vi "Write Extinction Data.vi"(8 "error in":errorcluster, 10 "CRDS Data in":refnum<class "CRDS Data.lvclass">, 11 "CRD File Obs in":refnum<class "CRD File Obs.lvclass">) -> (0 "error out":errorcluster, 3 "CRD File Obs out":refnum<class "CRD File Obs.lvclass">)   [LabVIEW 2015, in "CRD File Obs.lvclass"]
uses:
  CRD File Obs.lvclass
  Data/Main/CRDS Data.lvclass
  Data/Main/crd_data_enum.ctl
  Data/Cell/CRDS Cell Data.lvclass/CRDS Cell Data.ctl
  File IO/Class/File Observer.lvclass/File Observer.ctl
  Data/Cell/Read extParam.vi
  File IO/Class/Read File Ref.vi
  Data/Main/Read CellData.vi
  Data/Cell/CRDS Cell Data.lvclass
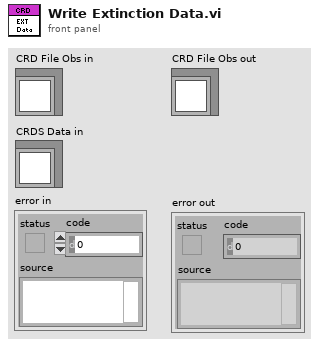
[diagram p1: front panel]
types:
  T1 = typedef "crd_data_enum.ctl" = enum8{"Time", "RHw", "TRH", "P", "Tmean", "RHsense", "TQ", "PQ", "Q", "Q0", "Qcal", "Qset", "extDilFac", "taucorr", "tau0corr", "stdevtau", "ext", "extCorr", "etau", "tau", "tau0", "Purge_Data", "NoData", "reserved", "Ttec", "Ang Exp", "Gamma", "filter", "fOverride", "notes", "max amp", "Tthermistor", "RhdilFac", "Psense", "TRHsense_bank", "RHsense_bank", "MFC_Data", "Thum", "ThumSP", "O3 Flow", "Pinlet Flow", "CLAP Flow", "O3 Add Valve", "O2 Valve", "O3 Cal"}
  T2 = enum16{"big-endian, network order", "native, host order", "little-endian"}
  T3 = typedef "extparam.ctl" = cluster{"Tau":sgl, "Tau0cor":sgl, "ext":sgl, "extCorr":sgl, "stdevTau":sgl, "eTau":sgl, "taucorr":sgl, "Tau0":sgl, "max":sgl}
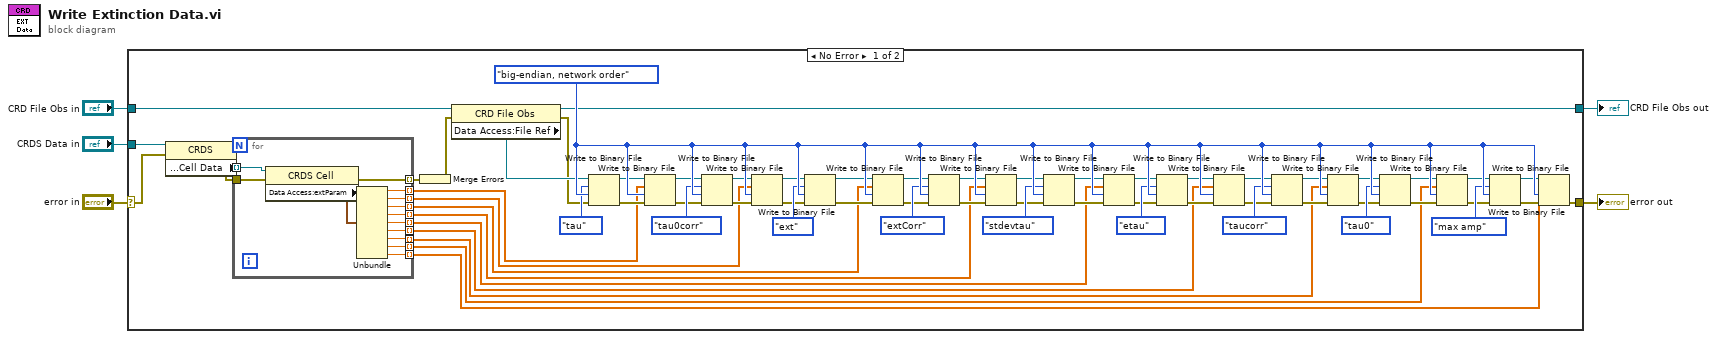
[diagram p0: block diagram]
diagram:
  n1 = case shown="No Error" "error in" {
    selector: "error in" -> [w67 w84]
    tunnel: [w7 w84] -> w4
    tunnel: [w6 w83] -> w2
    tunnel: "CRD File Obs in" -> [w11 w83]
    tunnel: "CRDS Data in" -> [w69 _]
    frame No Error {
      w65 = T2."big-endian, network order" ("byte order (0:big-endian, network order)")
      n2 = property class="CRDS"(reference=w69, error in=w67) -> (error out=w66:errorcluster, "Data Access:Cell Data"=w68:refnum<class "CRDS Cell Data.lvclass">[])  [unwired: 1 out]
      n3 = for {
        tunnel: w68 -> [w82] mode=indexing
        tunnel: w66 -> [w80]
        tunnel: [w79] -> w12 mode=indexing
        tunnel: [w78] -> w21 mode=indexing
        tunnel: [w77] -> w20 mode=indexing
        tunnel: [w76] -> w19 mode=indexing
        tunnel: [w75] -> w18 mode=indexing
        tunnel: [w74] -> w17 mode=indexing
        tunnel: [w73] -> w16 mode=indexing
        tunnel: [w72] -> w15 mode=indexing
        tunnel: [w71] -> w14 mode=indexing
        tunnel: [w70] -> w13 mode=indexing
        n4 = property class="CRDS Cell"(reference=w82, error in=w80) -> (error out=w79:errorcluster, "Data Access:extParam"=w81:T3)  [unwired: 1 out]
        n5 = Unbundle(w81) -> ("Tau"=w78:sgl, "Tau0cor"=w77:sgl, "ext"=w76:sgl, "extCorr"=w75:sgl, "stdevTau"=w74:sgl, "eTau"=w73:sgl, "taucorr"=w72:sgl, "Tau0"=w71:sgl, "max"=w70:sgl)
      }
      n6 = Merge Errors(w12) -> (w9:errorcluster)
      n7 = property class="CRD File Obs"(reference=w11, error in=w9) -> (reference out=w6:refnum<class "CRD File Obs.lvclass">, error out=w8:errorcluster, "Data Access:File Ref"=w10:refnum<file>)
      n8 = Write to Binary File(file (use dialog)=w10, data=crd_data_enum."tau" ("CRD_Data_Enum"), error in=w8, 9:w65) -> (refnum out=w42:refnum<file>, error out=w40:errorcluster)  [unwired: 2 in, 1 out]
      n9 = Write to Binary File(file (use dialog)=w42, data=w21, error in=w40, 9:w65) -> (refnum out=w43:refnum<file>, error out=w39:errorcluster)  [unwired: 2 in, 1 out]
      n10 = Write to Binary File(file (use dialog)=w43, data=crd_data_enum."tau0corr" ("CRD_Data_Enum"), error in=w39, 9:w65) -> (refnum out=w44:refnum<file>, error out=w38:errorcluster)  [unwired: 2 in, 1 out]
      n11 = Write to Binary File(file (use dialog)=w44, data=w20, error in=w38, 9:w65) -> (refnum out=w45:refnum<file>, error out=w37:errorcluster)  [unwired: 2 in, 1 out]
      n12 = Write to Binary File(file (use dialog)=w45, data=crd_data_enum."ext" ("CRD_Data_Enum"), error in=w37, 9:w65) -> (refnum out=w46:refnum<file>, error out=w36:errorcluster)  [unwired: 2 in, 1 out]
      n13 = Write to Binary File(file (use dialog)=w46, data=w19, error in=w36, 9:w65) -> (refnum out=w48:refnum<file>, error out=w35:errorcluster)  [unwired: 2 in, 1 out]
      n14 = Write to Binary File(file (use dialog)=w48, data=crd_data_enum."extCorr" ("CRD_Data_Enum"), error in=w35, 9:w65) -> (refnum out=w47:refnum<file>, error out=w34:errorcluster)  [unwired: 2 in, 1 out]
      n15 = Write to Binary File(file (use dialog)=w47, data=w18, error in=w34, 9:w65) -> (refnum out=w49:refnum<file>, error out=w33:errorcluster)  [unwired: 2 in, 1 out]
      n16 = Write to Binary File(file (use dialog)=w49, data=crd_data_enum."stdevtau" ("CRD_Data_Enum"), error in=w33, 9:w65) -> (refnum out=w50:refnum<file>, error out=w32:errorcluster)  [unwired: 2 in, 1 out]
      n17 = Write to Binary File(file (use dialog)=w50, data=w17, error in=w32, 9:w65) -> (refnum out=w31:refnum<file>, error out=w30:errorcluster)  [unwired: 2 in, 1 out]
      n18 = Write to Binary File(file (use dialog)=w31, data=crd_data_enum."etau" ("CRD_Data_Enum"), error in=w30, 9:w65) -> (refnum out=w29:refnum<file>, error out=w28:errorcluster)  [unwired: 2 in, 1 out]
      n19 = Write to Binary File(file (use dialog)=w29, data=w16, error in=w28, 9:w65) -> (refnum out=w27:refnum<file>, error out=w26:errorcluster)  [unwired: 2 in, 1 out]
      n20 = Write to Binary File(file (use dialog)=w27, data=crd_data_enum."taucorr" ("CRD_Data_Enum"), error in=w26, 9:w65) -> (refnum out=w24:refnum<file>, error out=w25:errorcluster)  [unwired: 2 in, 1 out]
      n21 = Write to Binary File(file (use dialog)=w24, data=w15, error in=w25, 9:w65) -> (refnum out=w23:refnum<file>, error out=w22:errorcluster)  [unwired: 2 in, 1 out]
      n22 = Write to Binary File(file (use dialog)=w23, data=crd_data_enum."tau0" ("CRD_Data_Enum"), error in=w22, 9:w65) -> (refnum out=w58:refnum<file>, error out=w59:errorcluster)  [unwired: 2 in, 1 out]
      n23 = Write to Binary File(file (use dialog)=w58, data=w14, error in=w59, 9:w65) -> (refnum out=w60:refnum<file>, error out=w61:errorcluster)  [unwired: 2 in, 1 out]
      n24 = Write to Binary File(file (use dialog)=w60, data=crd_data_enum."max amp" ("CRD_Data_Enum"), error in=w61, 9:w65) -> (refnum out=w63:refnum<file>, error out=w64:errorcluster)  [unwired: 2 in, 1 out]
      n25 = Write to Binary File(file (use dialog)=w63, data=w13, error in=w64, 9:w65) -> (error out=w7:errorcluster)  [unwired: 2 in, 2 out]
    }
    frame Error {
    }
  }
  "error out" <- w4
  "CRD File Obs out" <- w2
